vi "PH_Beckhoff_PPMA-Rods.declare digital OutputTags.vi"() -> (0 "Digital Outputs":T2, 1 "Description":string)   [LabVIEW 2014, in "PH_Beckhoff_PPMA-Rods.lvlib"]
uses:
  PH_Beckhoff_PPMA-Rods.lvlib
  PH_Beckhoff/PH_Beckhoff.Digital Outputs.ctl
  PH_Beckhoff_PPMA-Rods.Rods Tags.ctl
  PH_Beckhoff/PH_Beckhoff.lvlib
panel:
  in  "Digital Output Value":T1
  out "Right Size?":bool
  # "Let this VI run to check the size!"
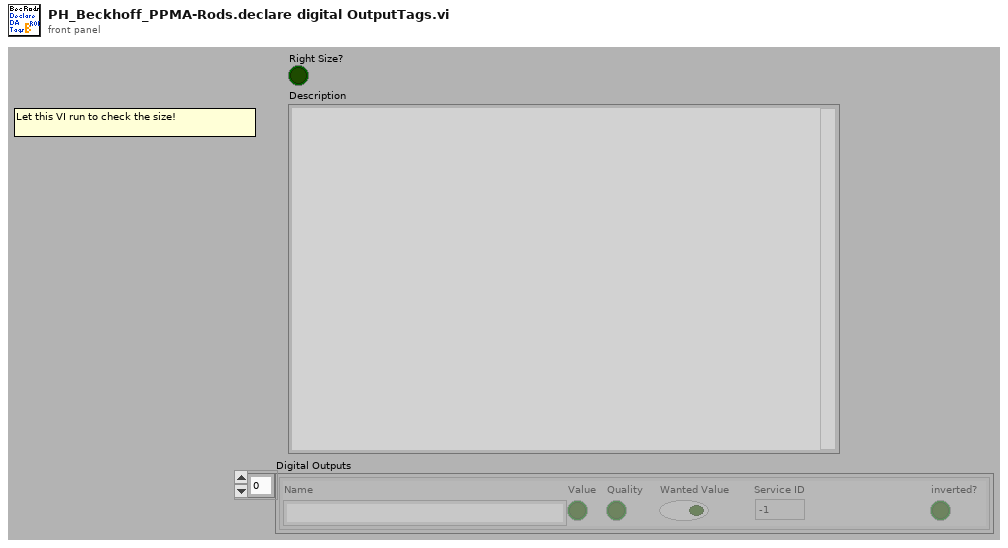
[diagram p1: front panel]
types:
  T1 = cluster{"Name":string, "Value":bool, "Quality":bool, "Wanted Value":bool, "Service ID":i32, "inverted?":bool}
  T2 = typedef "PH_Beckhoff.lvlib/PH_Beckhoff.Digital Outputs.ctl" = cluster{"Name":string, "Value":bool, "Quality":bool, "Wanted Value":bool, "Service ID":i32, "inverted?":bool}[]
  T3 = typedef "PH_Beckhoff_PPMA-Rods.lvlib/PH_Beckhoff_PPMA-Rods.Rods Tags.ctl" = enum16{"Rod-up", "earth-ok", "door-locked-K1", "door-locked-K2", "watervalve-closed", "Rods-Chain-A-up", "Rods-Chain-B-up", "HV-Warnlamp-orange", "HV-Warnlamp-green", "Status-Rods-PU-1", "Status-Rods-PU-2", "Status-Rods-PU-3", "Status-Rods-PU-4", "Status-Rods-PU-5", "Status-Rods-PU-6", "Status-Rods-PU-7", "Status-Rods-PU-8", "Status-Rods-PU-9", "Status-Rods-PU-10", "Status-Rods-FR", "Status-Rods-PILC"}
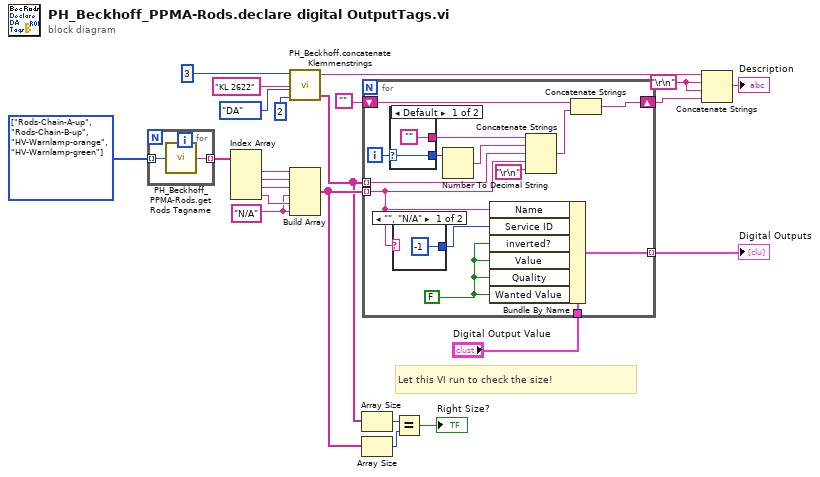
[diagram p0: block diagram]
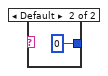
[diagram p2: hidden frame]
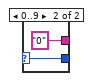
[diagram p3: hidden frame]
diagram:
  w2 = "N/A" ("element")
  w9 = T3[] [enum."Rods-Chain-A-up", enum."Rods-Chain-B-up", enum."HV-Warnlamp-orange", enum."HV-Warnlamp-green"] items=["Rod-up", "earth-ok", "door-locked-K1", "door-locked-K2", "watervalve-closed", "Rods-Chain-A-up", "Rods-Chain-B-up", "HV-Warnlamp-orange", "HV-Warnlamp-green", "Status-Rods-PU-1", "Status-Rods-PU-2", "Status-Rods-PU-3", "Status-Rods-PU-4", "Status-Rods-PU-5", "Status-Rods-PU-6", "Status-Rods-PU-7", "Status-Rods-PU-8", "Status-Rods-PU-9", "Status-Rods-PU-10", "Status-Rods-FR", "Status-Rods-PILC"]
  w23 = "\r\n"
  # "Let this VI run to check the size!"
  n1 = for {
    tunnel: w9 -> [w25] mode=indexing
    tunnel: [w24] -> w8 mode=indexing
    n2 = call "PH_Beckhoff_PPMA-Rods.get Rods Tagname.vi"("Rods Tag"=w25) -> ("Rods Tagname"=w24:string)
  }
  n3 = Index Array(array=w8) -> (element #1=w7:string, element #2=w5:string, element #3=w4:string, element #4=w3:string)  [unwired: 4 in]
  n4 = call "PH_Beckhoff.concatenate Klemmenstrings.vi"("# of In- or Outputs"=2, "Type"=enum16{"AE", "AA", "DE", "DA"}."DA", "Klemmenname"="KL 2622", "Quantity"=3 ("size(s)")) -> ("concatenated string array"=w1:string[], "\"<Type>: <Quantity> x <Klemmenname>\""=w10:string)  [unwired: 1 out]
  n5 = Build Array(w7, w5, w4, w2, w3, w2) -> (w6:string[])
  n6 = Array Size(array=w1) -> (size(s)=w21:i32)
  n7 = Array Size(array=w6) -> (size(s)=w19:i32)
  n8 = for {
    tunnel: w6 -> [w30] mode=indexing
    tunnel: w1 -> [w35] mode=indexing
    shift-right: [w33] -> w18
    shift-left: "" -> [w32]
    tunnel: "Digital Output Value" -> [w31]
    tunnel: [w28] -> w15 mode=indexing
    i -> [w39]
    w27 = FALSE ("Quality")
    n9 = case shown="Default" w39 {
      selector: w39 -> [w42 w45]
      tunnel: [w42 w45] -> w38
      tunnel: ["" "0"] -> w37
      frame Default {
      }
      frame 0..9 {
      }
    }
    n10 = case shown="\"\", \"N/A\"" w30 {
      tunnel: [-1 0] -> w29
      frame "", "N/A" {
      }
      frame Default {
      }
    }
    n11 = Number To Decimal String(number=w38) -> (decimal integer string=w36:string)  [unwired: 1 in]
    n12 = Bundle By Name(cluster=w31, "Name"=w30, "Service ID"=w29, "inverted?"=w27, "Value"=w27, "Quality"=w27, "Wanted Value"=w27) -> (w28:T1)
    n13 = Concatenate Strings(w37, w36, w35, w30, "\r\n") -> (w34:string)
    n14 = Concatenate Strings(w32, w34) -> (w33:string)
  }
  "Digital Outputs" <- w15
  n15 = Equal?(x=w21, y=w19) -> (x = y?=→"Right Size?":bool)
  n16 = Concatenate Strings(w10, w23, w23, w18) -> (→"Description":string)
